vi "LINX - Thumbstick Read.vi"() -> ()   [LabVIEW 2011, in "LVH-LINX.lvlib"]
doc: "Read the X-Y position of a thumbstick connected to a LINX device."
uses:
  vi.lib/LabVIEW Hacker/LINX/LVH-LINX.lvlib
  vi.lib/LabVIEW Hacker/LINX/Private/Type Defs/Thumbstick Data.ctl
panel:
  in  "Thumbstick Configuration":T1={"X Axis AI Channel"=0, "Y Axis AI Channel"=1, "Button DI Channel"=2}
  in  "Serial Port":refnum<visa-resource-name>
  in  "Stop Button":bool
  out "Loop Rate (Hz)":u32
  out "Thumbstick Data":T2
  out "XY Graph":cluster{dbl[], dbl[]}(graph)={[1.6583], [1.60678]}
  # "LINX Device Settings"
  # "Thumbstick \nConfiguration"
  # "Thumbstick Data"
  # "Thumbstick Example\n\nThis example demonstrates how read from a thumbstick using two analog input channels\nand one digital input channel.\n\nNote: This example is configured to use a serial interface but can easily be modified\nto use TCP or run on myRIO.\n\nInstructions\n1. Select the COM Port associated with the LIN Device.\n2. Select the AI Channels connected to the the X and Y axes and the DI Channel connected to the thumbstick button.\n3. Click the Run Arrow.\n4. Move the thumbstick and watch the graph update."
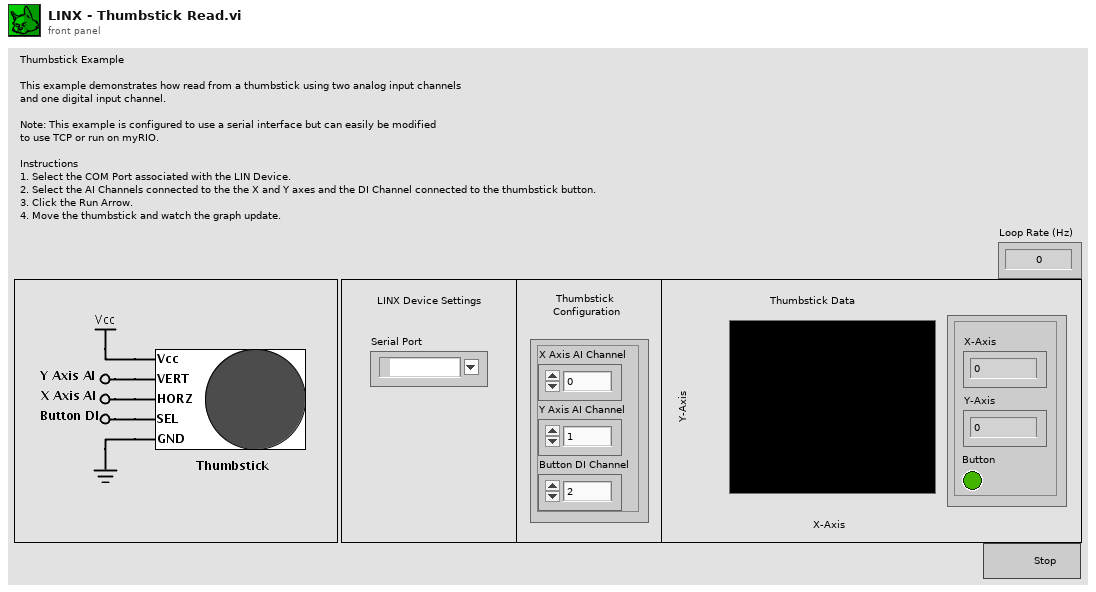
[diagram p1: front panel]
types:
  T1 = cluster{"X Axis AI Channel":u8, "Y Axis AI Channel":u8, "Button DI Channel":u8}
  T2 = typedef "LVH-LINX.lvlib/Thumbstick Data.ctl" = cluster{"X-Axis":dbl, "Y-Axis":dbl, "Button":bool}
  T3 = typedef "LVH-LINX.lvlib/LINX Ref.ctl" = cluster{"Platform":T4, "Interface":T5, "LINX Device Config":T6}
  T4 = typedef "LVH-LINX.lvlib/Platform.ctl" = enum16{"LINX", "myRIO"}
  T5 = typedef "LVH-LINX.lvlib/Interface.ctl" = enum16{"Serial", "TCP"}
  T6 = typedef "LVH-LINX.lvlib/Device.lvlib/LINX Device Config.ctl" = cluster{"Interface":T5, "COM Port":refnum<visa-resource-name>, "TCP Configuration":T7, "Device Family":u8, "Device ID":u8, "Device Name":string, "TCP Ref":refnum<k5>, "Channels":T8}
  T7 = typedef "LVH-LINX.lvlib/Device.lvlib/TCP Config.ctl" = cluster{"IP Address":string, "Port":u16}
  T8 = typedef "LVH-LINX.lvlib/Channels.ctl" = cluster{"DI Channels":u8[], "DO Channels":u8[], "AI":u8[], "AO":u8[], "PWM":u8[], "QE":u8[], "UART":u8[], "I2C 2":u8[], "SPI":u8[], "CAN":u8[], "AI Ref (V)":dbl, "AO Resolution (Bits)":u8, "AO Ref (V)":dbl}
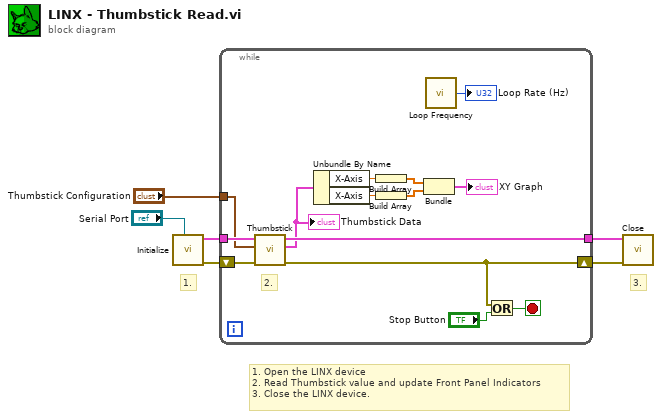
[diagram p0: block diagram]
diagram:
  # "3."
  # "1."
  # "1. Open the LINX device\n2. Read Thumbstick value and update Front Panel Indicators\n3. Close the LINX device."
  n1 = call "Initialize.vi"("Serial Port"="Serial Port") -> ("Error Out"=w3:errorcluster, "LINX Ref"=w4:T3)  [unwired: 8 in, 1 out]
  n2 = while {
    shift-right: [w7] -> w6
    shift-left: w3 -> [w16]
    tunnel: w4 -> [w17]
    tunnel: [w15] -> w2
    tunnel: "Thumbstick Configuration" -> [w14]
    stop <- w20 stop-if-true
    # "2."
    n3 = call "Thumbstick.vi"("Error In"=w16, "Thumbstick Configuration"=w14, "LINX Resource"=w17) -> ("Error Out"=w7:errorcluster, "Thumbstick Data"=w8:T2, "LINX Resource"=w15:T3)  [unwired: 6 in]
    "Thumbstick Data" <- w8
    n4 = Unbundle By Name(w8) -> ("X-Axis"=w9:dbl, "X-Axis"=w10:dbl)
    n5 = Build Array(w9) -> (w11:dbl[])
    n6 = Build Array(w10) -> (w12:dbl[])
    n7 = Bundle(w11, w12) -> (→"XY Graph":cluster{dbl[], dbl[]})  [unwired: 1 in]
    n8 = call "Loop Frequency.vi"() -> ("Loop Rate (Hz)"=→"Loop Rate (Hz)":u32)
    n9 = Or(x=w7, y="Stop Button") -> (x .or. y?=w20:bool)
  }
  n10 = call "Close.vi"("Error In"=w6, "LINX Resource"=w2) -> ()  [unwired: 8 in, 2 out]
